vi "Host Main.vi"() -> ()   [LabVIEW 2017]
doc: "This application launches and executes the Tag Bus Data framework configuration for the specified target alias. This is a simple example of the framework API functions, but may also be a suitable starting point for a Host UI or Thick Client that is running a local version of the framework."
uses:
  <vilib>/NI/Module Execution Interface/Engine Runtime/Execution States.ctl
  <vilib>/NI/Module Execution Interface/Engine Runtime/Fault.ctl
  <vilib>/NI/Tag Bus Module Framework/runtime/error classification.ctl
  Utilities/Controlword_Commands.ctl
  <vilib>/NI/STM/TCP/Read Meta Data (TCP Ref).vi
  <vilib>/NI/STM/TCP/Get Connection Reference (TCP).vi
  <vilib>/NI/STM/TCP/Read Meta Data (TCP Clst).vi
  <vilib>/NI/STM/TCP/Write Message (TCP).vi
  <vilib>/NI/STM/TCP/Read Message (TCP).vi
  <vilib>/userdefined/High Color/nirio_resource_hc.ctl
  <vilib>/NI/Module Execution Interface/Engine Runtime/Engine Runtime Interface.lvclass
  <vilib>/NI/DCAF/Tag Editor Core/Framework Configuration Classes/target runtime/PL_Target Runtime.lvclass
  <vilib>/NI/Tag Bus Module Framework/FPGA manager/FPGA manager.lvlib
  <vilib>/rvi/interface/nirviOpenFPGA/nirviOpenFPGA.xnode
  <vilib>/NI/Tag Bus Module Framework/FPGA manager/methods.ctl
  <vilib>/NI/Tag Bus Module Framework/runtime/TBM module execution interface.lvclass
  <vilib>/NI/STM/NI STM.lvlib
  Utilities/WordManipulationLibrary.lvlib
panel:
  in  "Positions":dbl[](array[numeric])
  in  "Velocity":dbl=1000.0
  in  "Acceleration":dbl=10000.0
  in  "Acceleration Jerk":dbl=1000.0
  in  "StraightLineMove":bool
  in  "StateChange":bool
  in  "Device Control Command":T1
  in  "StateName":string="StateChange"
  in  "Target IP Address":string="localhost"
  in  "Network Stop":bool
  out "error  out":errorcluster
  in  "configuration file path":path
  in  "target alias":string="PC"
  out "engine status":T5(array[cluster])
  in  "Engine_Stop":bool
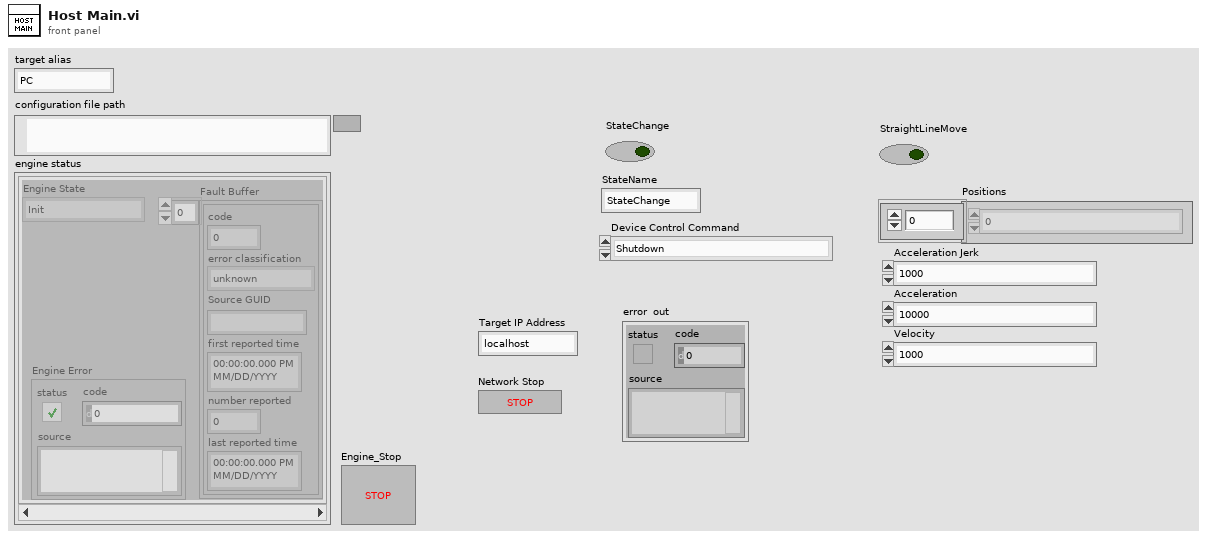
[diagram p1: front panel]
types:
  T1 = typedef "WordManipulationLibrary.lvlib/Controlword_Commands.ctl" = enum16{"Shutdown", "Switch On", "Disable Voltage", "Quick Stop", "Disable Op", "Enable Op", "Fault Reset", "Error"}
  T2 = typedef "Engine Runtime Interface.lvclass/Execution States.ctl" = enum16{"Init", "Pre-Operational", "Safe-Operational", "Operational", "Stopped"}
  T3 = typedef "Engine Runtime Interface.lvclass/Fault.ctl" = cluster{"code":i32, "error classification":T4, "Source GUID":string, "first reported time":timestamp, "number reported":u32, "last reported time":timestamp}
  T4 = typedef "TBM module execution interface.lvclass/error classification.ctl" = enum16{"unknown", "none", "trivial", "recoverable", "critical"}
  T5 = cluster{"Engine State":T2, "Fault Buffer":T3[], "Engine Error":errorcluster}[]
  T6 = typedef "FPGA manager.lvlib/methods.ctl" = enum16{"initialize bitfile", "cache bitfile", "locate bitfile", "close bitfile", "clear manager"}
  T7 = typedef "nirio_resource_hc.ctl" = tag
  T8 = typedef "NI STM.lvlib/TCP Connection Info.ctl" = cluster{"connection ID":refnum<k5>, "meta data":T9[]}
  T9 = typedef "NI STM.lvlib/MetaDataElement.ctl" = string
  T10 = cluster{"Engine State":T2, "Fault Buffer":T3[], "Engine Error":errorcluster}
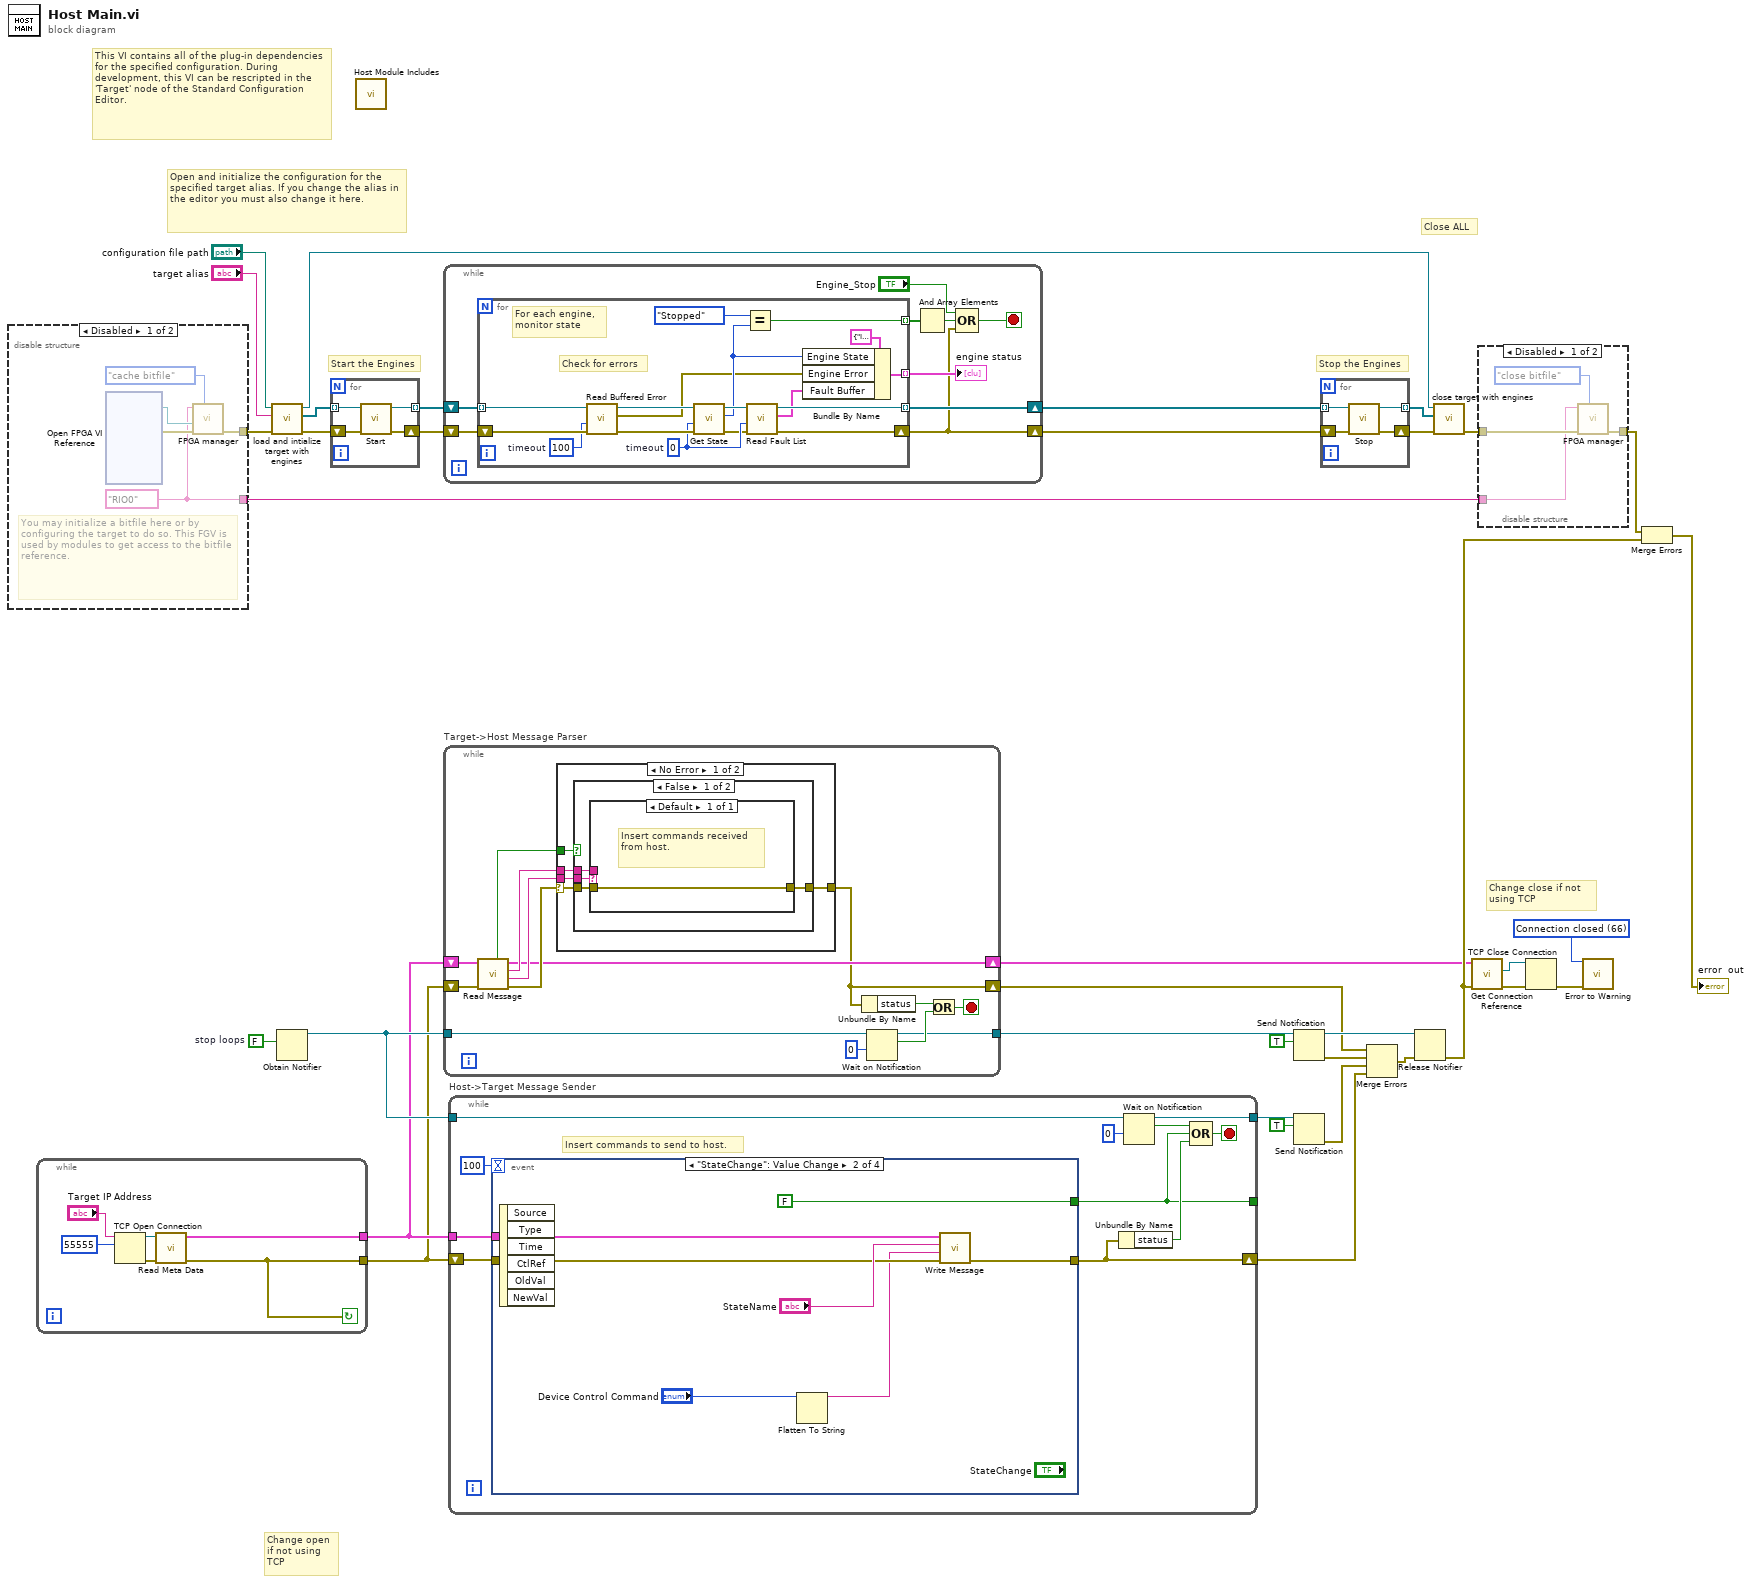
[diagram p0: block diagram]
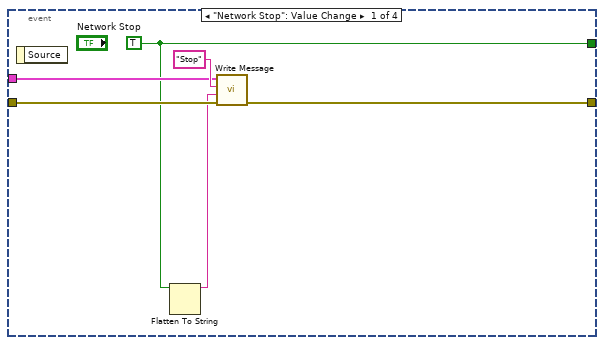
[diagram p2: hidden frame]
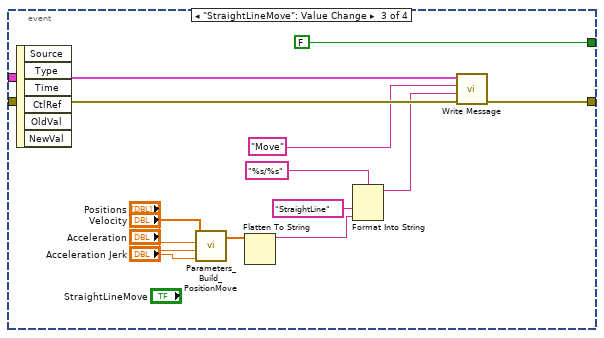
[diagram p3: hidden frame]
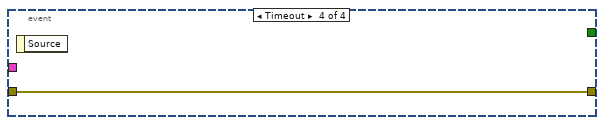
[diagram p4: hidden frame]
diagram:
  w5 = FALSE  # stop loops
  w19 = 66 items=["No Error", "Argument Error", "Memory Full", "Out of Zone", "End of File", "File Already Open", "Generic File IO Error", "File Not Found", "File Permission Error", "Disk Full", "Duplicate Path", "Too Many Files Open", "Not Enabled", "Resource File Not Found", "Cannot Add Resource", "Resource Not Found", "Image Not Found", "Image Memory Error", "Pen Does Not Exist", "Config Bad Type", "Config Token Not Found", "Config Parse Error", "Config Memory Error", "Bad External Code Format", "Bad External Code Offset", "External Code Not Present", "Null Window", "Destroy Window Mixup", "Null Menu", "Print Aborted", "Bad Print Record", "Print Driver Error", "Windows Error During Print", "Memory Error During Print", "Print Dialog Error", "Generic Print Error", "Invalid Device Refnum", "Device Not Found", "Device Parameter Error", "Device Unit Error", "Can't Open Device", "Device Call Aborted", "Generic Error", "Cancelled By User", "Object ID Too Low", "Object ID Too High", "Object Not In Heap", "Unknown Heap", "Bad DefProc ID", "DefProc Not In Table", "Message Out Of Range", "Null Method", "Unknown Message", "Manager Call Not Supported", "Bad address", "Connection In progress", "Connection timed out", "Connection is already in progress", "Network attribute not supported", "Network error", "Address in use", "System out of memory", "Connection aborted", "Connection refused", "Connection is not connected", "Connection is already connected", "Connection closed", "Initialize error (interapplication manager)", "Bad occurrence", "Wait on unbound occurrence handler", "Occurrence queue overflow", "Bad path", "Semaphore not signaled", "Unrecognized type (interapplication manager)"] ("1st Error to Convert")
  # "Change close if not using TCP"
  # "Change open if not using TCP"
  # "Start the Engines"
  # "Open and initialize the configuration for the specified target alias. If you change the alias in the editor you must also change it here."
  # "Close ALL"
  # "Stop the Engines"
  # "This VI contains all of the plug-in dependencies for the specified configuration. During development, this VI can be rescripted in the 'Target' node of the Standard Configuration Editor."
  n1 = disable-structure shown="Disabled" {
    disable-tunnel: [w41 _] -> w26
    disable-tunnel: [w37 _] -> w25
    frame Disabled {
      w37 = T7 "RIO0" ("RIO resource")
      # "You may initialize a bitfile here or by configuring the target to do so. This FGV is used by modules to get access to the bitfile reference."
      n2 = xnode "Open FPGA VI Reference"() -> ("FPGA VI Reference Out"=w39:refnum<k20>, "error out"=w40:errorcluster)  [unwired: 2 in]
      n3 = call <vilib>:"FPGA manager.vi"("action"=methods."cache bitfile", "error in"=w40, "bitfile to cache"=w39, "RIO resource"=w37) -> ("error out"=w41:errorcluster)  [unwired: 5 in, 2 out]
    }
    frame Enabled {
    }
  }
  n4 = while {
    tunnel: [w47] -> w4
    tunnel: [w42] -> w3
    stop <- w42 continue-if-true
    n5 = TCP Open Connection(address="Target IP Address", remote port or service name=u16 55555 ("remote port")) -> (connection ID=w46:refnum<k5>, error out=w45:errorcluster)  [unwired: 1 in, 2 out]
    n6 = call-poly <vilib>:"Read Meta Data.vi"("error in"=w45, "connection ID"=w46) -> ("error out"=w42:errorcluster, "connection info out"=w47:T8)  [unwired: 1 in, 7 out]
  }
  n7 = call <vilib>:"load and intialize target with engines.vi"("error in"=w26, "target alias"="target alias", "file path"="configuration file path") -> ("error out"=w33:errorcluster, "engine runtime interfaces"=w32:refnum<class "Engine Runtime Interface.lvclass">[], "target runtime"=w29:refnum<class "PL_Target Runtime.lvclass">)  [unwired: 6 in]
  n8 = Obtain Notifier(notification data type=w5) -> (notifier out=w8:refnum<notifier>)  [unwired: 3 in, 2 out]
  n9 = for {
    tunnel: [w51] -> w36 mode=indexing
    tunnel: w32 -> [w48] mode=indexing
    shift-right: [w50] -> w21
    shift-left: w33 -> [w49]
    n10 = call-dynamic "Start.vi"("error in"=w49, "Engine Runtime Interface in"=w48) -> ("error out"=w50:errorcluster, "Engine Runtime Interface out"=w51:refnum<class "Engine Runtime Interface.lvclass">)  [unwired: 8 in]
  }
  n11 = call "Host Module Includes.vi"() -> ()  [unwired: 12 in]
  n12 = while {
    shift-right: [w58] -> w35
    shift-left: w36 -> [w60]
    shift-right: [w52] -> w34
    shift-left: w21 -> [w59]
    stop <- w56 stop-if-true
    n13 = for {
      tunnel: w60 -> [w77] mode=indexing
      tunnel: [w69] -> w58 mode=indexing
      tunnel: [w72] -> w54 mode=indexing
      shift-right: [w68] -> w52
      shift-left: w59 -> [w76]
      tunnel: [w64] -> w55 mode=indexing
      w67 = 0  # timeout
      w71 = 100  # timeout
      # "For each engine, \nmonitor state"
      # "Check for errors"
      n14 = call-dynamic "Read Buffered Error.vi"("error in"=w76, "timeout in ms (0)"=w71, "Engine Runtime Interface in"=w77) -> ("error out"=w74:errorcluster, "Engine Error"=w62:errorcluster, "Engine Runtime Interface out"=w75:refnum<class "Engine Runtime Interface.lvclass">)  [unwired: 6 in]
      n15 = call-dynamic "Get State.vi"("error in"=w74, "timeout (-1)"=w67, "Engine Runtime Interface in"=w75) -> ("error out"=w61:errorcluster, "Engine State"=w66:T2, "Engine Runtime Interface out"=w70:refnum<class "Engine Runtime Interface.lvclass">)  [unwired: 6 in]
      n16 = Equal?(x=Execution_States."Stopped" ("Engine State"), y=w66) -> (x = y?=w72:bool)
      n17 = call-dynamic "Read Fault List.vi"("error in"=w61, "timeout (-1)"=w67, "Engine Runtime Interface in"=w70) -> ("error out"=w68:errorcluster, "faults"=w65:T3[], "Engine Runtime Interface out"=w69:refnum<class "Engine Runtime Interface.lvclass">)  [unwired: 6 in]
      n18 = Bundle By Name(cluster=T10 {"Engine State"=enum."Init", "Fault Buffer"=[], "Engine Error"={"status"=FALSE, "code"=0, "source"=""}}, "Engine State"=w66, "Engine Error"=w62, "Fault Buffer"=w65) -> (w64:T10)
    }
    "engine status" <- w55
    n19 = And Array Elements(Boolean array=w54) -> (logical AND=w53:bool)
    n20 = Compound Arithmetic op=OR("Engine_Stop", w53, w52) -> (w56:bool)
  }
  n21 = while "Target->Host Message Parser" {
    shift-right: [w78] -> w2
    shift-left: w3 -> [w90]
    tunnel: w8 -> [w84]
    tunnel: [w80] -> w6
    shift-right: [w85] -> w18
    shift-left: w4 -> [w91]
    stop <- w81 stop-if-true
    n22 = call-poly <vilib>:"Read Message.vi"("error in"=w90, "connection info in"=w91) -> ("error out"=w86:errorcluster, "name"=w89:T9, "data string"=w88:string, "connection info out"=w85:T8, "timed out?"=w87:bool)  [unwired: 3 in, 2 out]
    n23 = case shown="No Error" w86 {
      selector: w86 -> [w93 w103]
      tunnel: w89 -> [w96 _]
      tunnel: w88 -> [w95 _]
      tunnel: w87 -> [w94 _]
      tunnel: [w92 w103] -> w78
      frame No Error {
        n24 = case shown="False" w94 {
          tunnel: w96 -> [w97 _]
          tunnel: w95 -> [w100 _]
          tunnel: w93 -> [w99 w102]
          tunnel: [w98 w102] -> w92
          frame False {
            n25 = case shown="Default" w97 {
              tunnel: w100 -> [_]
              tunnel: w99 -> [w101]
              tunnel: [w101] -> w98
              frame Default {
                # "Insert commands received from host."
              }
            }
          }
          frame True {
          }
        }
      }
      frame Error {
      }
    }
    n26 = Unbundle By Name(w78) -> ("status"=w79:bool)
    n27 = Wait on Notification(notifier=w84, timeout in ms (-1)=0) -> (notifier out=w80:refnum<notifier>, notification=w82:bool)  [unwired: 2 in, 2 out]
    n28 = Or(x=w79, y=w82) -> (x .or. y?=w81:bool)
  }
  n29 = while "Host->Target Message Sender" {
    shift-right: [w106] -> w11
    shift-left: w3 -> [w114]
    tunnel: w4 -> [w113]
    tunnel: w8 -> [w110]
    tunnel: [w107] -> w9
    tunnel: [w104] -> _
    stop <- w108 stop-if-true
    # "Insert commands to send to host."
    n30 = event shown="[1] \"StateChange\": Value Change" {
      selector: _ -> [_ _ _ _]
      dyn-events: _ -> [_ _ _ _]
      timeout: 100 -> [_ _ _ _]
      tunnel: w113 -> [w119 w126 w141 _]
      tunnel: w114 -> [w118 w125 w140 w142]
      tunnel: [w116 FALSE ("stop") FALSE ("stop") _] -> w104
      tunnel: [w115 w122 w138 w142] -> w106
      event "Network Stop": Value Change {
        w116 = TRUE ("stop")
        n31 = event-data() -> ()  [unwired: 2 out]
        n32 = Flatten To String(anything=w116) -> (data string=w117:string)  [unwired: 2 in, 3 out]
        n33 = call-poly <vilib>:"Write Message.vi"("error in"=w118, "data"=w117, "name"="Stop" ("Name"), "connection info in"=w119) -> ("error out"=w115:errorcluster)  [unwired: 1 in, 6 out]
      }
      event "StateChange": Value Change {
        n34 = event-data() -> ()  [unwired: 7 out]
        n35 = Flatten To String(anything="Device Control Command") -> (data string=w124:string)  [unwired: 2 in, 3 out]
        n36 = call-poly <vilib>:"Write Message.vi"("error in"=w125, "data"=w124, "name"="StateName", "connection info in"=w126) -> ("error out"=w122:errorcluster)  [unwired: 1 in, 6 out]
      }
      event "StraightLineMove": Value Change {
        n37 = event-data() -> ()  [unwired: 7 out]
        n38 = call "Parameters_Build_PositionMove.vi"("Acceleration Jerk"="Acceleration Jerk", "Acceleration"="Acceleration", "Velocity"="Velocity", "Positions"="Positions") -> ("Parameters"=w133:dbl[])  [unwired: 7 in]
        n39 = Flatten To String(anything=w133) -> (data string=w132:string)  [unwired: 2 in, 3 out]
        n40 = Format Into String(format string="%s/%s", "StraightLine" ("input 1"), w132) -> (resulting string=w134:string)  [unwired: 2 in, 1 out]
        n41 = call-poly <vilib>:"Write Message.vi"("error in"=w140, "data"=w134, "name"="Move", "connection info in"=w141) -> ("error out"=w138:errorcluster)  [unwired: 1 in, 6 out]
      }
      event Timeout {
        n42 = event-data() -> ()  [unwired: 2 out]
      }
    }
    n43 = Unbundle By Name(w106) -> ("status"=w105:bool)
    n44 = Wait on Notification(notifier=w110, timeout in ms (-1)=0) -> (notifier out=w107:refnum<notifier>, notification=w112:bool)  [unwired: 2 in, 2 out]
    n45 = Compound Arithmetic op=OR(w112, w104, w105) -> (w108:bool)
  }
  n46 = Send Notification(notification=TRUE, notifier=w6) -> (notifier out=w14:refnum<notifier>, error out=w13:errorcluster)  [unwired: 1 in]
  n47 = Send Notification(notification=TRUE, notifier=w9) -> (error out=w12:errorcluster)  [unwired: 1 in, 1 out]
  n48 = for {
    tunnel: w35 -> [w146] mode=indexing
    shift-right: [w143] -> w28
    shift-left: w34 -> [w145]
    tunnel: [w144] -> w30 mode=indexing
    n49 = call-dynamic "Stop.vi"("error in"=w145, "Engine Runtime Interface in"=w146) -> ("error out"=w143:errorcluster, "Engine Runtime Interface out"=w144:refnum<class "Engine Runtime Interface.lvclass">)  [unwired: 8 in]
  }
  n50 = Merge Errors(w2, w13, w12, w11) -> (w15:errorcluster)
  n51 = Release Notifier(notifier=w14, error in (no error)=w15) -> (error out=w22:errorcluster)  [unwired: 1 in, 2 out]
  n52 = call <vilib>:"close target with engines.vi"("error in"=w28, "Engine Runtime Interfaces"=w30, "Target Runtime"=w29) -> ("error out"=w24:errorcluster)  [unwired: 8 in]
  n53 = call-poly <vilib>:"Get Connection Reference.vi"("error in"=w22, "connection info in"=w18) -> ("error out"=w17:errorcluster, "connection ID out"=w16:refnum<k5>)  [unwired: 8 out]
  n54 = disable-structure shown="Disabled" {
    disable-tunnel: [w149 w151] -> w23
    disable-tunnel: w24 -> [w150 w151]
    disable-tunnel: w25 -> [w147 _]
    frame Disabled {
      n55 = call <vilib>:"FPGA manager.vi"("action"=methods."close bitfile", "error in"=w150, "RIO resource"=w147) -> ("error out"=w149:errorcluster)  [unwired: 6 in, 2 out]
    }
    frame Enabled {
    }
  }
  n56 = TCP Close Connection(connection ID=w16, error in (no error)=w17) -> (error out=w20:errorcluster)  [unwired: 2 out]
  n57 = call <vilib>:"Error to Warning.vi"("1st Error to Convert"=w19, "error in"=w20) -> ()  [unwired: 3 in, 11 out]
  n58 = Merge Errors(w23, w22) -> (→"error  out":errorcluster)
